vi "PS Control.vi"() -> ()   [LabVIEW 2016]
panel:
  out "Value Changed":bool
  in  "stop":bool
  in  "Slew Rate [T/Min]":dbl=1.0 caption="(7.055) Max)" min=0.001 max=50.0 step=0.01 format="%.3f"
  in  "Setpoint [T]":dbl caption="(34.68) Max)" min=-34.679602421022246 max=34.679602421022246 format="%.5f"
  in  "Pause":bool
  out "Field [T]":dbl caption="Current [kA]" format="%.5f"
  in  "Units":enum32{"tesla", "kAmps"}(radio) caption="tesla            kAmps"
  in  "Ramp":bool
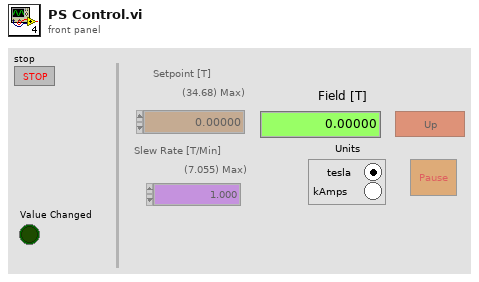
[diagram p1: front panel]
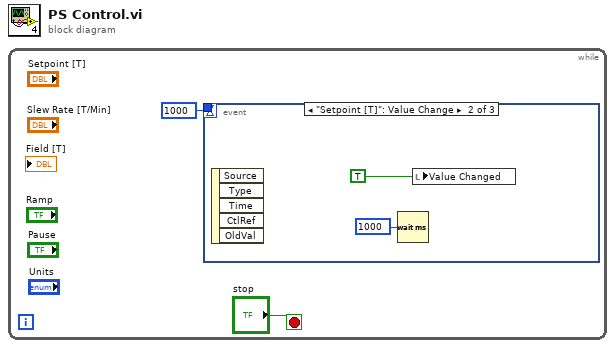
[diagram p0: block diagram]
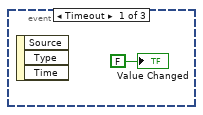
[diagram p2: hidden frame]
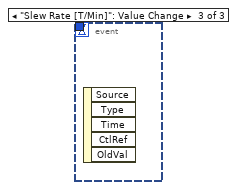
[diagram p3: hidden frame]
diagram:
  n1 = while {
    stop <- "stop" stop-if-true
    n2 = event shown="[1] \"Setpoint [T]\": Value Change" {
      selector: _ -> [_ _ _]
      dyn-events: _ -> [_ _ _]
      timeout: 1000 -> [_ _ w6]
      tunnel: [_ _ w6] -> _
      event Timeout {
        n3 = event-data() -> ()  [unwired: 1 in, 3 out]
        "Value Changed" <- FALSE ("Value Changed")
      }
      event "Setpoint [T]": Value Change {
        n4 = event-data() -> ()  [unwired: 1 in, 5 out]
        n5 = Wait (ms)(milliseconds to wait=u32 1000) -> ()  [unwired: 1 out]
        n6 = local write "Value Changed"(TRUE ("Value Changed 2")) -> ()
      }
      event "Slew Rate [T/Min]": Value Change {
        n7 = event-data() -> ()  [unwired: 1 in, 5 out]
      }
    }
  }
